vi "Autonomous Independent.vi"() -> ()   [LabVIEW 2016]
doc: "This VI is called when autonomous begins, and will automatically be terminated when autonomous ends. You can carry out timed or sensor driven robot movement independently without needing to return to the caller."
uses:
  2_8_17/Auto_Action.ctl
  <vilib>/Rock Robotics/Network Tables/NT Read Number.vi
  2_11_17/Systems/Global 1.vi
panel:
  out "In Range?":bool=TRUE
  out "Auto Mode":dbl=7.0
  in  "Auton_Modes":T2(array[cluster])=[{"Actions"=[{"Effort"=0.55, "Duration"=3.5, "Action"=enum."Nothing", "Encoder"=0.0, "Condition"=FALSE}, {"Effort"=0.0, "Duration"=0.0, "Action"=enum."Nothing", "Encoder"=0.0, "Condition"=FALSE}]}, {"Actions"=[{"Effort"=0.0, "Duration"=0.1, "Action"=enum."Gear1", "Encoder"=6.462, "Condition"=FALSE}, {"Effort"=0.0, "Duration"=0.1, "Action"=enum."Nothing", "Encoder"=0.0, "Condition"=FALSE}, {"Effort"=0.25, "Duration"=1.0, "Action"=enum."Nothing", "Encoder"=38.0, "Condition"=FALSE}, {"Effort"=0.0, "Duration"=0.1, "Action"=enum."Nothing", "Encoder"=0.0, "Condition"=FALSE}, {"Effort"=0.25, "Duration"=0.0, "Action"=enum."Nothing", "Encoder"=57.0, "Condition"=FALSE}, {"Effort"=-0.25, "Duration"=0.0, "Action"=enum."Nothing", "Encoder"=0.0, "Condition"=FALSE}, {"Effort"=1.0, "Duration"=0.0, "Action"=enum."Nothing", "Encoder"=0.0, "Condition"=FALSE}, {"Effort"=0.25, "Duration"=0.0, "Action"=enum."Nothing", "Encoder"=0.0, "Condition"=FALSE}]}, {"Actions"=[{"Effort"=0.0, "Duration"=0.1, "Action"=enum."Drive Encoder Reset", "Encoder"=0.0, "Condition"=FALSE}, {"Effort"=0.0, "Duration"=1.0, "Action"=enum."Gyro Reset", "Encoder"=0.0, "Condition"=FALSE}, {"Effort"=0.3, "Duration"=2.0, "Action"=enum."Drive", "Encoder"=88.0, "Condition"=TRUE}, {"Effort"=1.0, "Duration"=1.0, "Action"=enum."Gear0", "Encoder"=0.0, "Condition"=FALSE}, {"Effort"=1.0, "Duration"=1.0, "Action"=enum."Gear0", "Encoder"=0.0, "Condition"=FALSE}, {"Effort"=1.0, "Duration"=0.5, "Action"=enum."Nothing", "Encoder"=0.0, "Condition"=FALSE}, {"Effort"=0.0, "Duration"=0.0, "Action"=enum."Drive Encoder Reset", "Encoder"=0.0, "Condition"=FALSE}, {"Effort"=0.3, "Duration"=0.5, "Action"=enum."Nothing", "Encoder"=24.0, "Condition"=TRUE}, {"Effort"=0.0, "Duration"=0.0, "Action"=enum."Nothing", "Encoder"=0.0, "Condition"=FALSE}, {"Effort"=-0.2, "Duration"=0.75, "Action"=enum."Drive", "Encoder"=24.0, "Condition"=FALSE}, {"Effort"=0.0, "Duration"=0.0, "Action"=enum."Drive Encoder Reset", "Encoder"=0.0, "Condition"=FALSE}, {"Effort"=-0.25, "Duration"=0.0, "Action"=enum."Nothing", "Encoder"=12.0, "Condition"=FALSE}]}, {"Actions"=[{"Effort"=0.0, "Duration"=0.1, "Action"=enum."Drive Encoder Reset", "Encoder"=6.462, "Condition"=FALSE}, {"Effort"=0.0, "Duration"=0.1, "Action"=enum."Gyro Reset", "Encoder"=0.0, "Condition"=FALSE}, {"Effort"=-0.25, "Duration"=1.0, "Action"=enum."Drive", "Encoder"=6.462, "Condition"=FALSE}, {"Effort"=0.0, "Duration"=0.1, "Action"=enum."Gyro Reset", "Encoder"=0.0, "Condition"=FALSE}, {"Effort"=-0.25, "Duration"=0.0, "Action"=enum."Turn", "Encoder"=57.0, "Condition"=FALSE}, {"Effort"=-0.25, "Duration"=0.0, "Action"=enum."Drive", "Encoder"=7.5, "Condition"=FALSE}, {"Effort"=-1.0, "Duration"=0.0, "Action"=enum."Gear0", "Encoder"=0.0, "Condition"=FALSE}, {"Effort"=0.25, "Duration"=0.0, "Action"=enum."Drive", "Encoder"=3.0, "Condition"=FALSE}]}, {"Actions"=[{"Effort"=0.0, "Duration"=0.1, "Action"=enum."Drive Encoder Reset", "Encoder"=6.462, "Condition"=FALSE}, {"Effort"=0.0, "Duration"=0.1, "Action"=enum."Gyro Reset", "Encoder"=0.0, "Condition"=FALSE}, {"Effort"=-0.25, "Duration"=1.0, "Action"=enum."Drive", "Encoder"=72.0, "Condition"=FALSE}, {"Effort"=0.0, "Duration"=0.1, "Action"=enum."Gyro Reset", "Encoder"=0.0, "Condition"=FALSE}, {"Effort"=-0.25, "Duration"=2.0, "Action"=enum."Turn", "Encoder"=57.0, "Condition"=FALSE}, {"Effort"=-0.25, "Duration"=0.0, "Action"=enum."Drive", "Encoder"=36.0, "Condition"=FALSE}, {"Effort"=-1.0, "Duration"=0.0, "Action"=enum."Gear0", "Encoder"=0.0, "Condition"=FALSE}, {"Effort"=0.25, "Duration"=0.0, "Action"=enum."Drive", "Encoder"=24.0, "Condition"=FALSE}]}, {"Actions"=[{"Effort"=0.0, "Duration"=0.1, "Action"=enum."Vision Correction", "Encoder"=0.0, "Condition"=FALSE}, {"Effort"=0.0, "Duration"=0.1, "Action"=enum."Nothing", "Encoder"=0.0, "Condition"=FALSE}, {"Effort"=0.25, "Duration"=1.0, "Action"=enum."Nothing", "Encoder"=6.462, "Condition"=FALSE}, {"Effort"=1.0, "Duration"=0.1, "Action"=enum."Nothing", "Encoder"=0.0, "Condition"=FALSE}, {"Effort"=0.25, "Duration"=0.0, "Action"=enum."Nothing", "Encoder"=57.0, "Condition"=FALSE}, {"Effort"=0.25, "Duration"=0.0, "Action"=enum."Nothing", "Encoder"=7.5, "Condition"=FALSE}, {"Effort"=1.0, "Duration"=0.0, "Action"=enum."Nothing", "Encoder"=0.0, "Condition"=FALSE}, {"Effort"=-0.25, "Duration"=0.0, "Action"=enum."Nothing", "Encoder"=3.0, "Condition"=FALSE}]}, {"Actions"=[{"Effort"=0.0, "Duration"=0.1, "Action"=enum."Drive Encoder Reset", "Encoder"=0.0, "Condition"=FALSE}, {"Effort"=0.0, "Duration"=0.1, "Action"=enum."Gyro Reset", "Encoder"=0.0, "Condition"=FALSE}, {"Effort"=0.25, "Duration"=5.0, "Action"=enum."Drive", "Encoder"=60000.0, "Condition"=TRUE}, {"Effort"=0.75, "Duration"=1.0, "Action"=enum."Nothing", "Encoder"=0.0, "Condition"=FALSE}, {"Effort"=0.0, "Duration"=1.0, "Action"=enum."Nothing", "Encoder"=0.0, "Condition"=FALSE}, {"Effort"=0.0, "Duration"=0.0, "Action"=enum."Nothing", "Encoder"=0.0, "Condition"=FALSE}]}, {"Actions"=[{"Effort"=0.0, "Duration"=0.5, "Action"=enum."Drive Encoder Reset", "Encoder"=0.0, "Condition"=FALSE}, {"Effort"=0.55, "Duration"=4.25, "Action"=enum."Gyro Reset", "Encoder"=0.0, "Condition"=FALSE}, {"Effort"=0.5, "Duration"=0.0, "Action"=enum."Drive", "Encoder"=43.0, "Condition"=FALSE}, {"Effort"=0.3, "Duration"=1.3, "Action"=enum."Turn", "Encoder"=0.0, "Condition"=TRUE}, {"Effort"=0.3, "Duration"=1.0, "Action"=enum."Drive Encoder Reset", "Encoder"=12.0, "Condition"=FALSE}, {"Effort"=0.3, "Duration"=0.5, "Action"=enum."Vision Correction", "Encoder"=5.0, "Condition"=FALSE}, {"Effort"=0.3, "Duration"=1.0, "Action"=enum."Drive", "Encoder"=18.5, "Condition"=TRUE}, {"Effort"=1.0, "Duration"=0.0, "Action"=enum."Gear0", "Encoder"=0.0, "Condition"=FALSE}, {"Effort"=-0.3, "Duration"=0.0, "Action"=enum."Drive", "Encoder"=30.0, "Condition"=FALSE}, {"Effort"=-0.3, "Duration"=1.3, "Action"=enum."Turn", "Encoder"=0.0, "Condition"=FALSE}, {"Effort"=0.4, "Duration"=0.0, "Action"=enum."Drive", "Encoder"=10.0, "Condition"=FALSE}]}, {"Actions"=[{"Effort"=0.0, "Duration"=0.0, "Action"=enum."Nothing", "Encoder"=0.0, "Condition"=FALSE}, {"Effort"=0.0, "Duration"=0.0, "Action"=enum."Nothing", "Encoder"=0.0, "Condition"=FALSE}, {"Effort"=0.0, "Duration"=0.0, "Action"=enum."Gyro Reset", "Encoder"=0.0, "Condition"=FALSE}]}]
  # "Nothing"
  # "Boiler Right Right side gear"
  # "Middle Gear"
  # "Boiler Right Left Side Gear"
  # "Boiler Left RightSide Gear"
  # "Boiler Left Left Side Gear"
  # "Drive"
  # "Vision Correction"
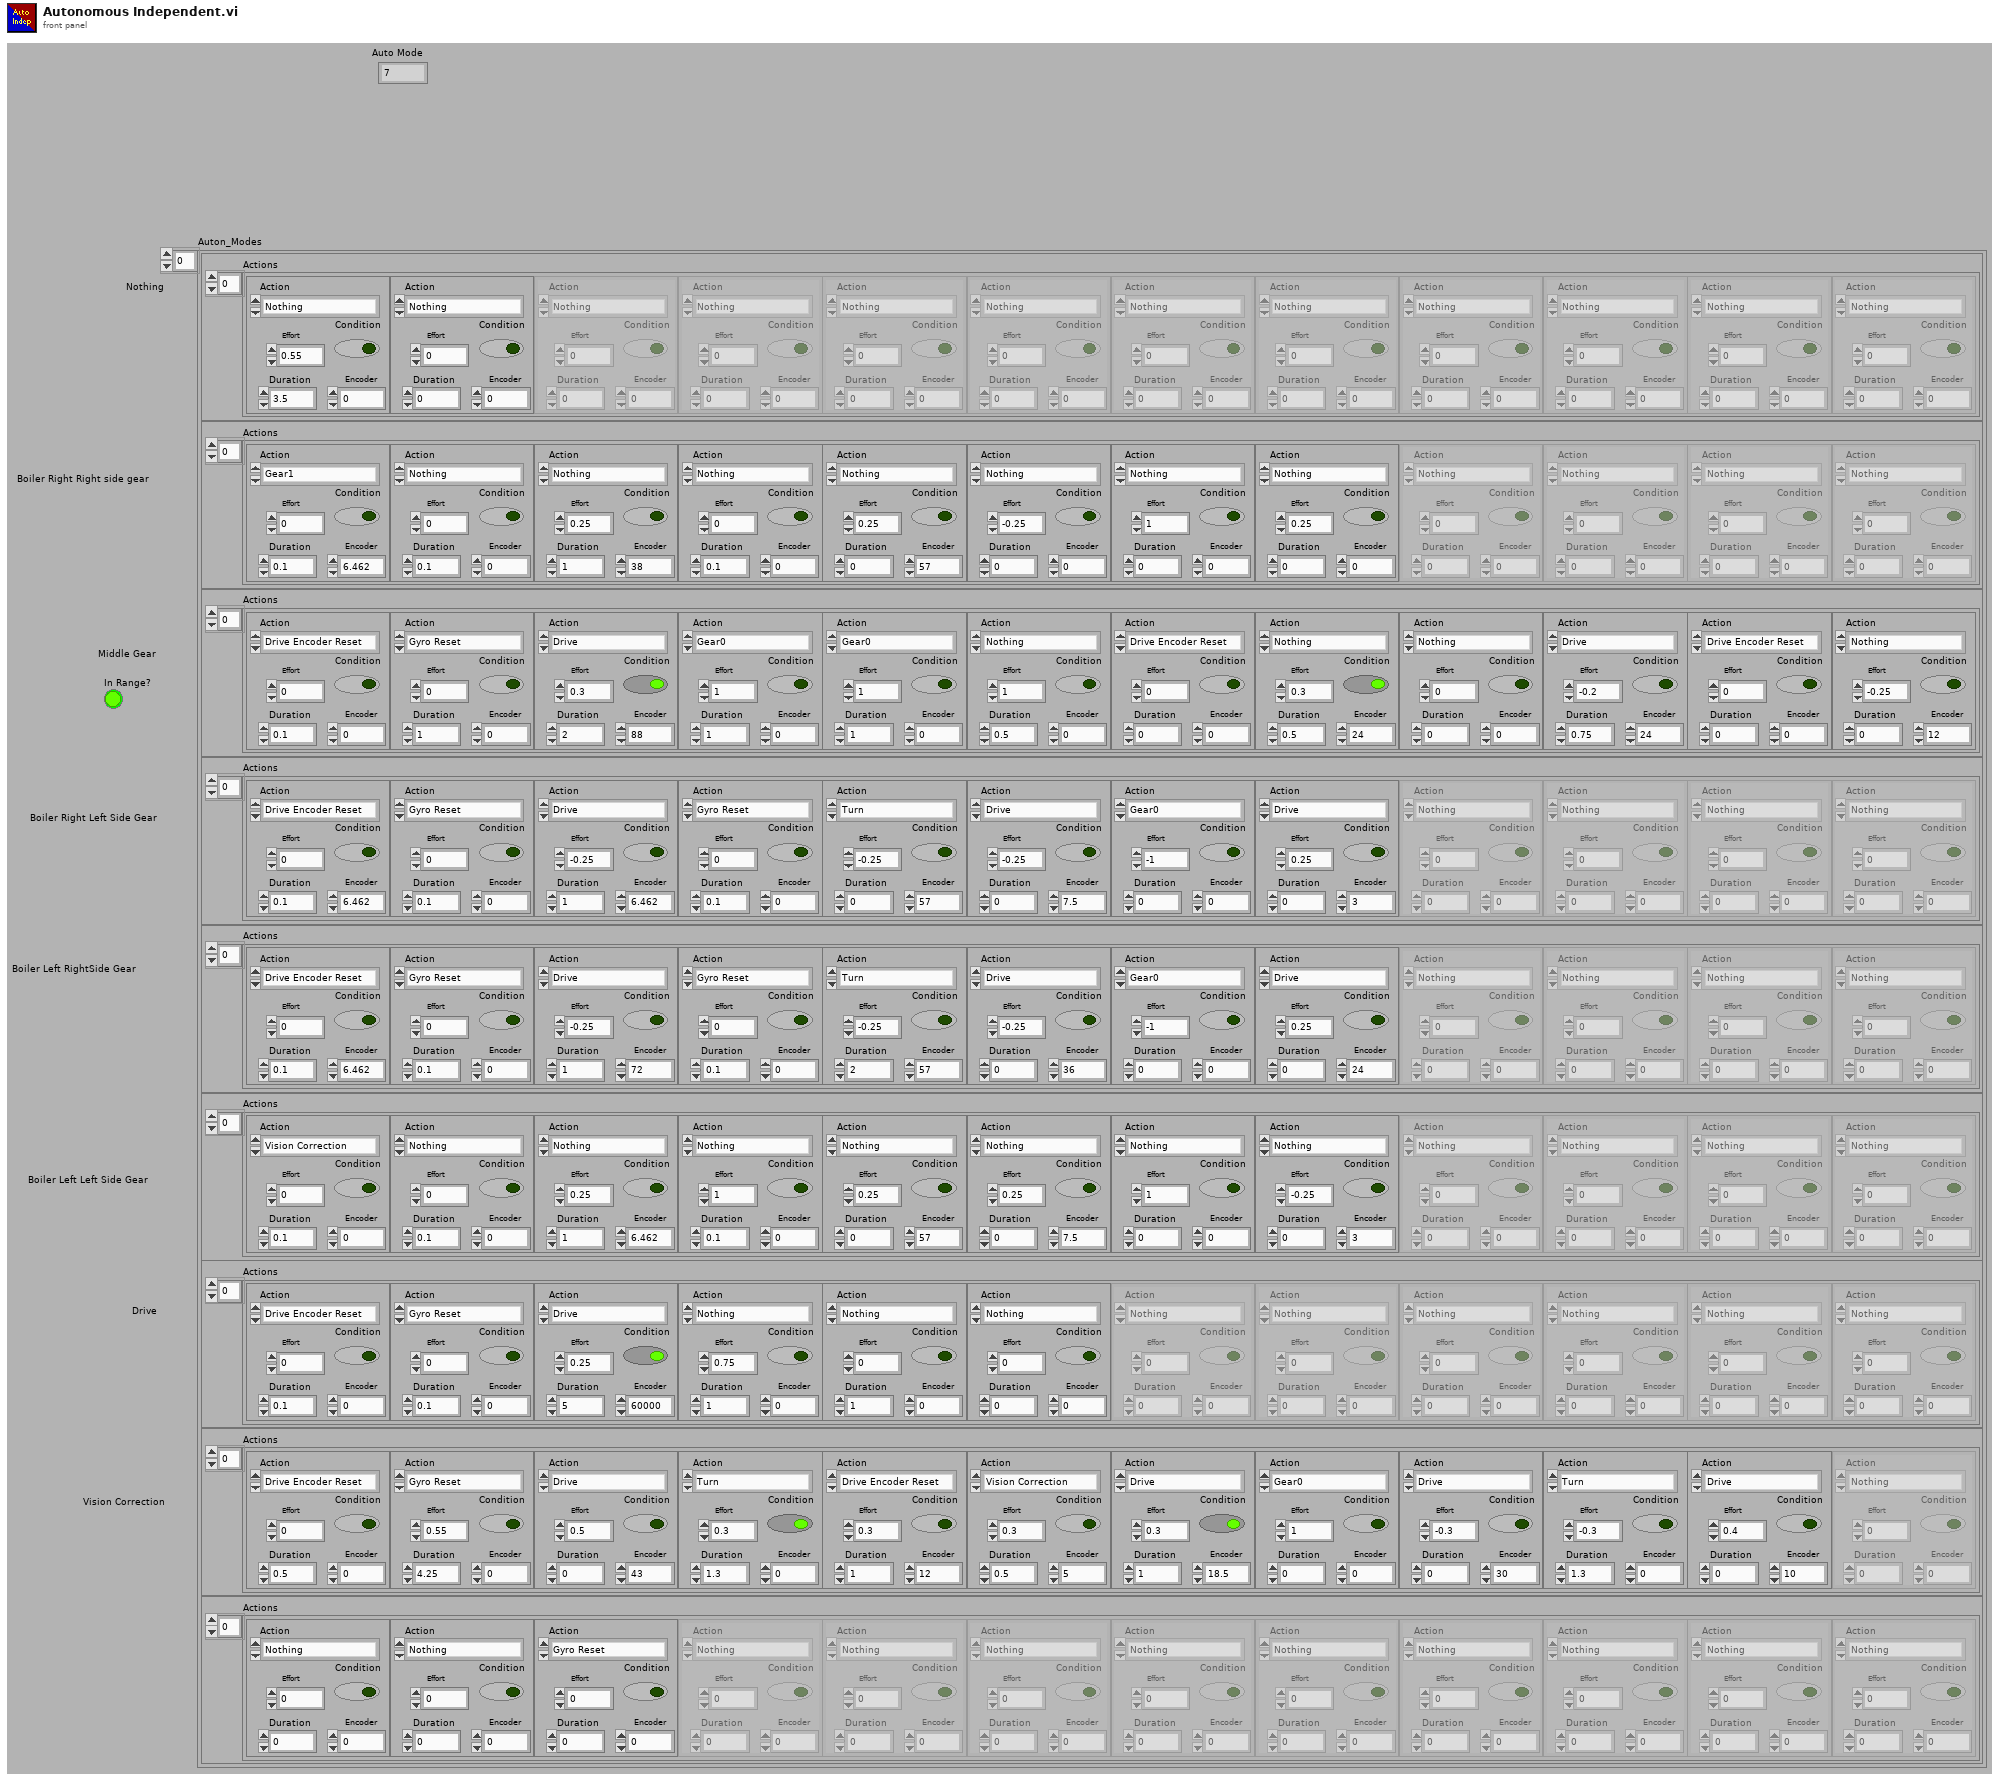
[diagram p1: front panel]
types:
  T1 = typedef "Auto_Action.ctl" = enum16{"Nothing", "Drive", "Vision Correction", "Turn", "Gear0", "Gear1", "Climb", "Intake", "Index", "Shoot", "Test", "Drive Encoder Reset", "Gyro Reset"}
  T2 = cluster{"Actions":cluster{"Effort":dbl, "Duration":dbl, "Action":T1, "Encoder":dbl, "Condition":bool}[]}[]
  T3 = cluster{"Actions":cluster{"Effort":dbl, "Duration":dbl, "Action":T1, "Encoder":dbl, "Condition":bool}[]}
  T4 = cluster{"Effort":dbl, "Duration":dbl, "Action":T1, "Encoder":dbl, "Condition":bool}[]
  T5 = typedef "WPI_MotorControlDeviceRef.ctl" = cluster{"DeviceStatus":errorcluster, "Type":T6, "PWM":cluster{"PWM Channel":T7, "DeadBand":T8}, "CAN":cluster{"Device Number":u8, "SetOutput VI Ref":variant, "GetOutput VI Ref":variant, "Enable VI Ref":variant, "Disable VI Ref":variant, "Data":variant}, "Invert":bool}
  T6 = typedef "WPI_MotorControlType.ctl" = enum16{"PWM", "CAN"}
  T7 = typedef "FPGA_DIOPWMChannel.ctl" = enum8{"PWM 0", "PWM 1", "PWM 2", "PWM 3", "PWM 4", "PWM 5", "PWM 6", "PWM 7", "PWM 8", "PWM 9", "PWM MXP 0", "PWM MXP 1", "PWM MXP 2", "PWM MXP 3", "PWM MXP 4", "PWM MXP 5", "PWM MXP 6", "PWM MXP 7", "PWM MXP 8", "PWM MXP 9", "Invalid"}
  T8 = typedef "WPI_PWMDeadband.ctl" = cluster{"Name":string, "maxPositivePwm":i32, "minPositivePwm":i32, "centerPwm":i32, "maxNegativePwm":i32, "minNegativePwm":i32, "angularRange":u16}
  T9 = typedef "WPI_CANTalonSRX_GlobalStatus.ctl" = cluster{"Applied Throttle":dbl, "Module Enabled":bool, "CAN Error":errorcluster, "Closed Loop Error":dbl, "Forward Limit Switch Closed":bool, "Reverse Limit Switch Closed":bool, "Sensor Position":dbl, "Sensor Velocity":dbl, "Current":dbl, "Sticky Fault - Over Temp":bool, "Sticky Fault - Under Voltage":bool, "Sticky Fault - Forward Limit":bool, "Sticky Fault - Reverse Limit":bool, "Sticky Fault - Forward Soft Limit":bool, "Sticky Fault - Reverse Soft Limit":bool, "Brake is Enabled":bool, "Encoder Position":dbl, "Encoder Velocity":dbl, "Encoder Index Count":dbl, "Encoder A Pin State":bool, "Encoder B Pin State":bool, "Encoder Index Pin State":bool, "Analog In":dbl, "Analog In Velocity":dbl, "Temperature (C)":dbl, "Battery Voltage":dbl, "Control 5 Is Supported":bool, "Current Profile Slot Select":dbl, "Pos Div 8":bool, "Vel Div 4":bool, "Pulse Width Position":i32, "Pulse Width Velocity":i32, "Pulse Width Rise To Rise (us)":i32, "Pulse Width Rise To Fall (us)":i32, "Mot Prof Active Is Under Run":bool, "Mot Prof Active Has Under Run":bool, "Mot Prof Active Is Last":bool, "Mot Prof Active Velocity Only":bool, "Mot Prof Active Is Valid":bool, "Mot Prof Buffer Is Full":bool, "Mot Prof Active Profile Slot Select":i32, "Mot Prof NextID":i32, "Mot Prof Count":i32, "Mot Prof Active Velocity":dbl, "Mot Prof Active Position":dbl, "Mot Prof Output Enable":i32}
  T10 = typedef "WPI_GyroDevRef.ctl" = cluster{"DevStatus":errorcluster, "Analog Channel":T11, "Offset":dbl, "Gain (VoltsPerDegree/Second)":dbl, "Gyro Type":enum16{"Analog", "XRS450"}, "Handle":i32, "SPI Bus":T12, "Device Found":bool, "Sample Rate":dbl, "Calibrate On Open":bool}
  T11 = typedef "FPGA_AIChannel.ctl" = enum8{"AI 0", "AI 1", "AI 2", "AI 3", "AI MXP 0", "AI MXP 1", "AI MXP 2", "AI MXP 3", "Invalid"}
  T12 = typedef "spi_bus.ctl" = enum16{"SPI On-Board, CS0", "SPI On-Board, CS1", "SPI On-Board, CS2", "SPI On-Board, CS3", "SPI MXP", "Invalid"}
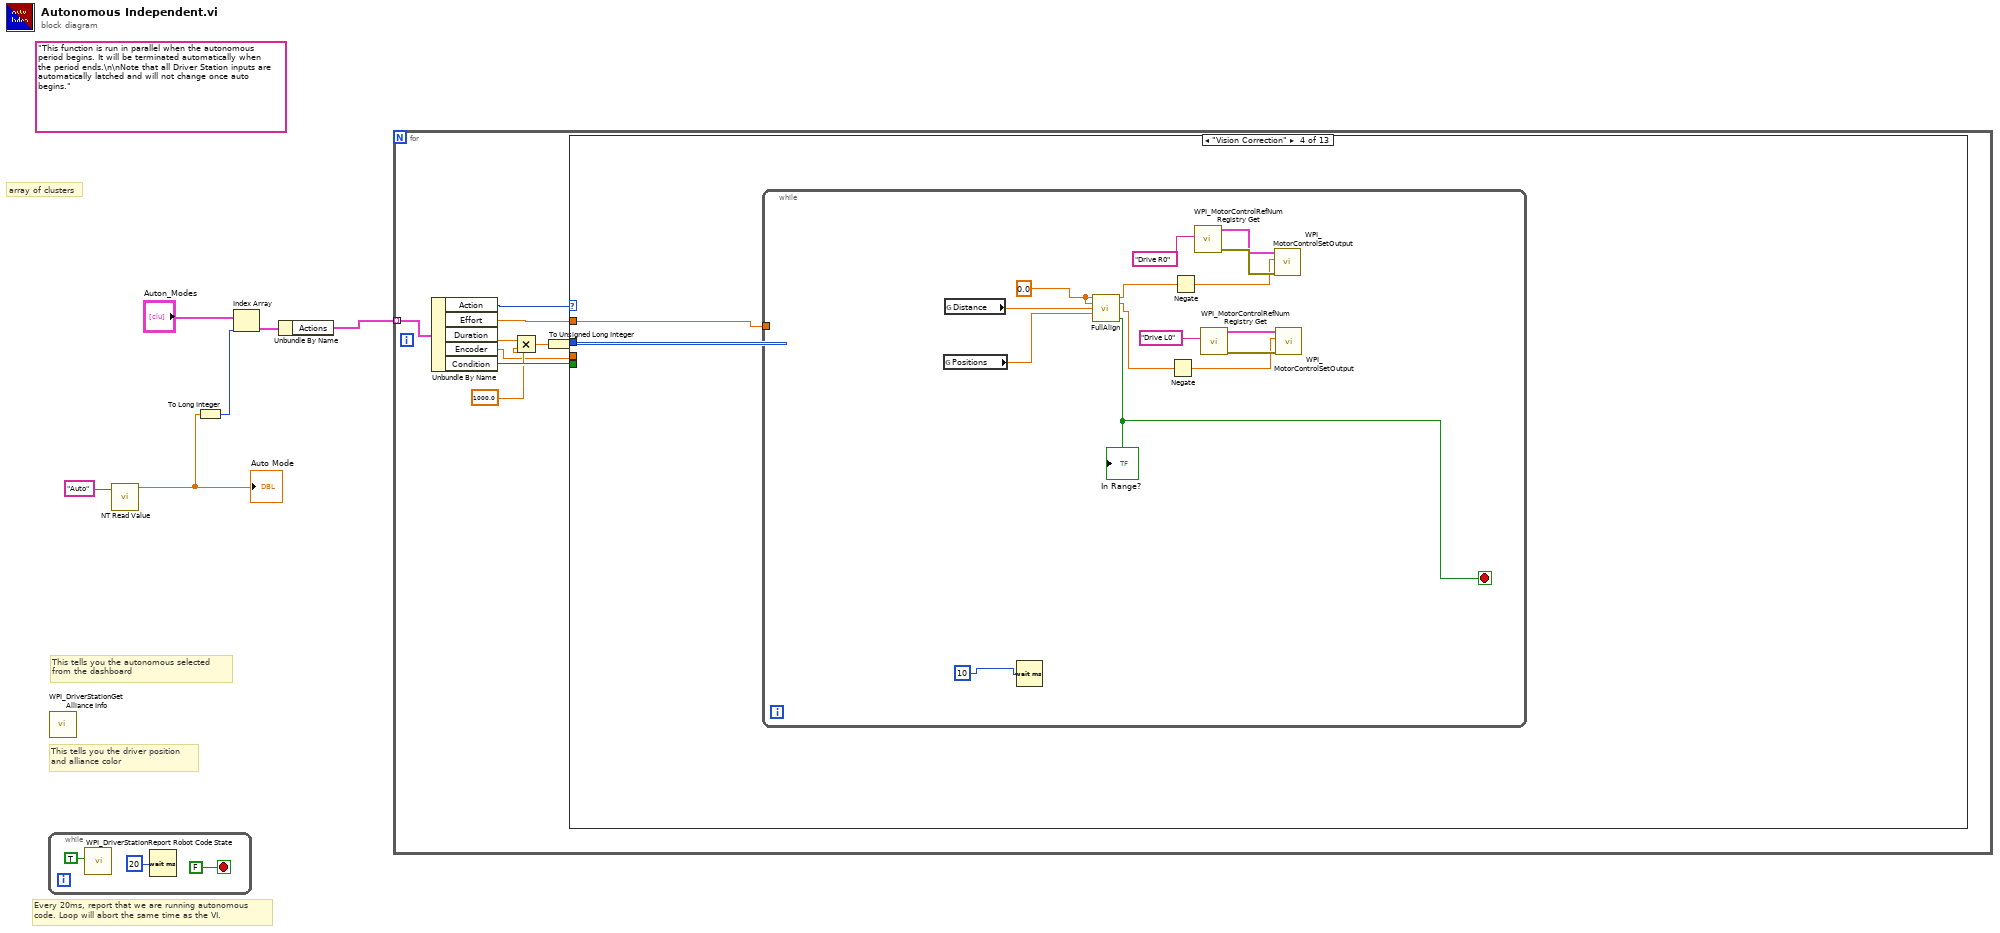
[diagram p0: block diagram]
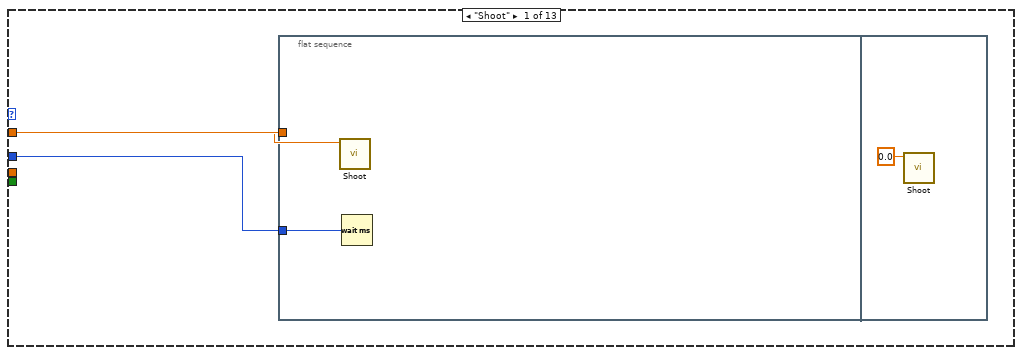
[diagram p2: hidden frame]
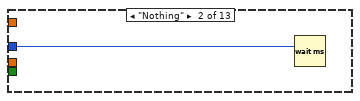
[diagram p3: hidden frame]
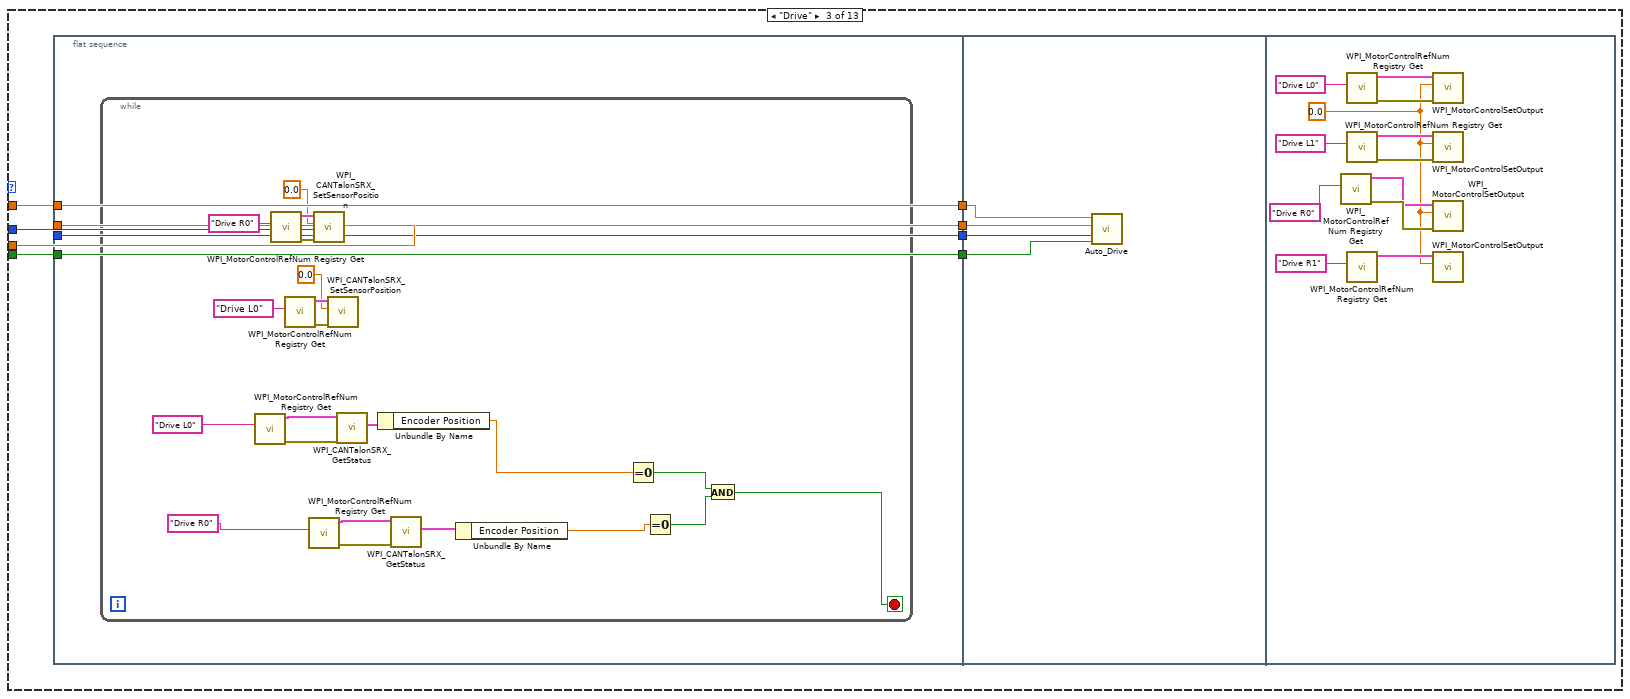
[diagram p4: hidden frame]
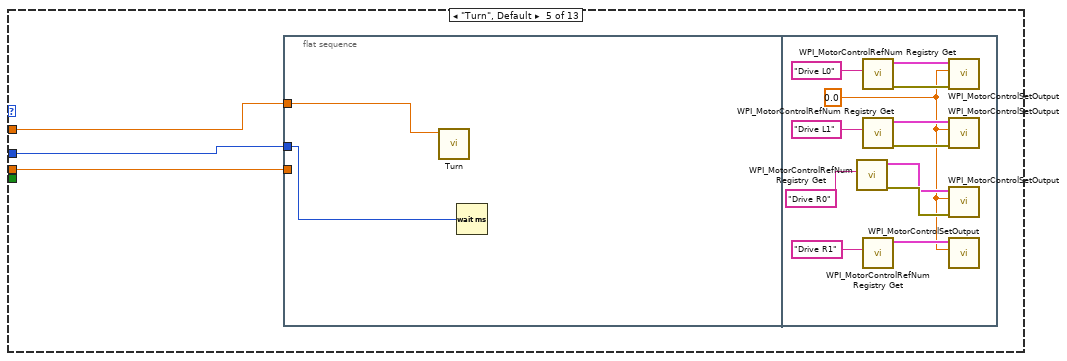
[diagram p5: hidden frame]
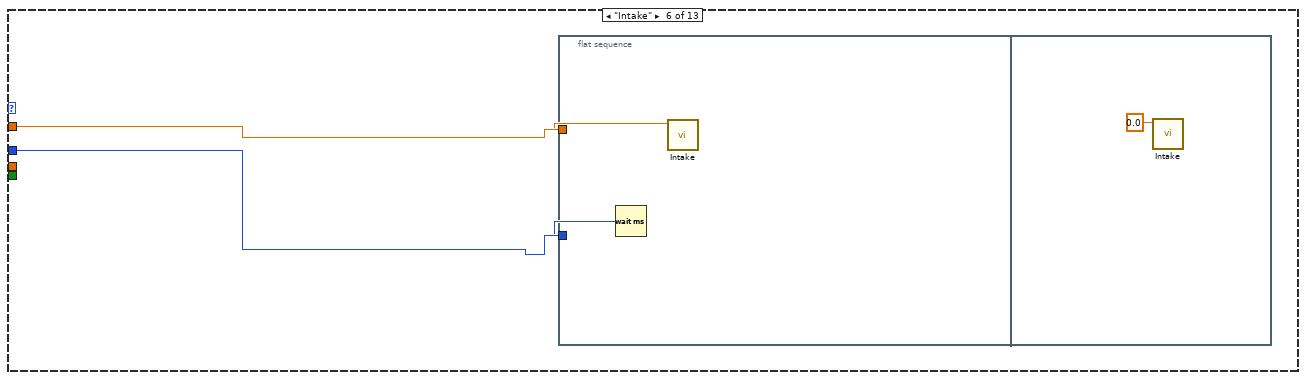
[diagram p6: hidden frame]
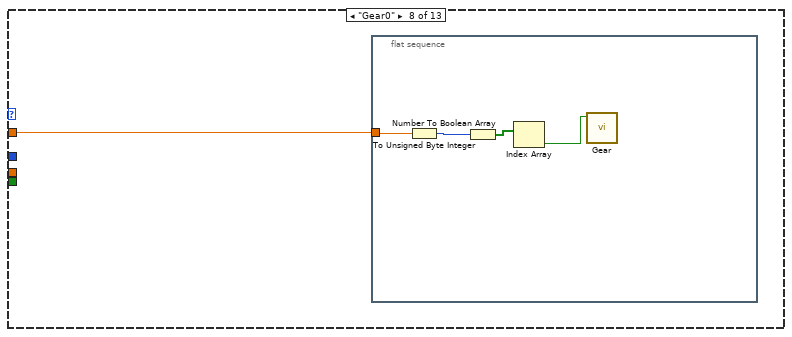
[diagram p8: hidden frame]
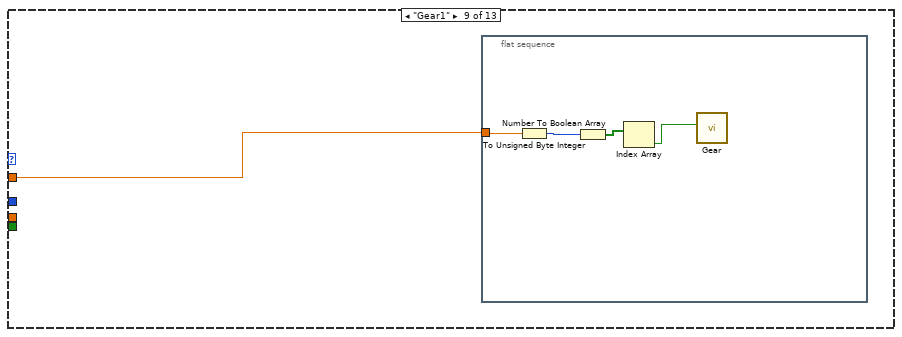
[diagram p9: hidden frame]
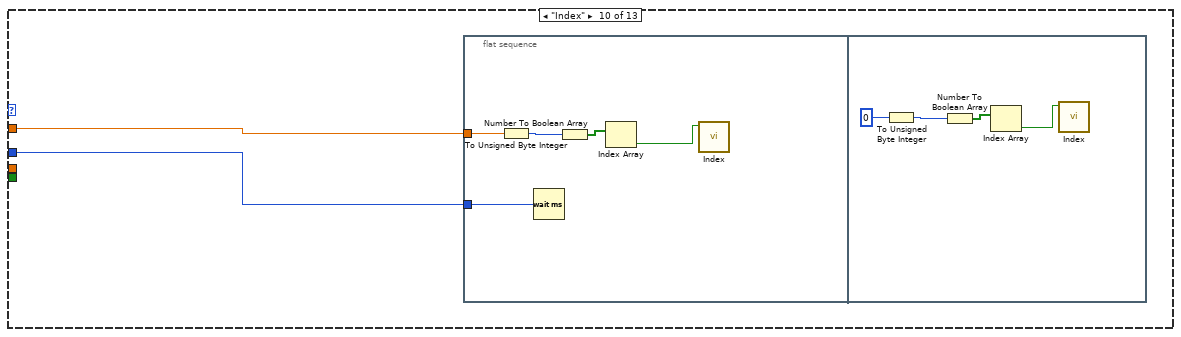
[diagram p10: hidden frame]
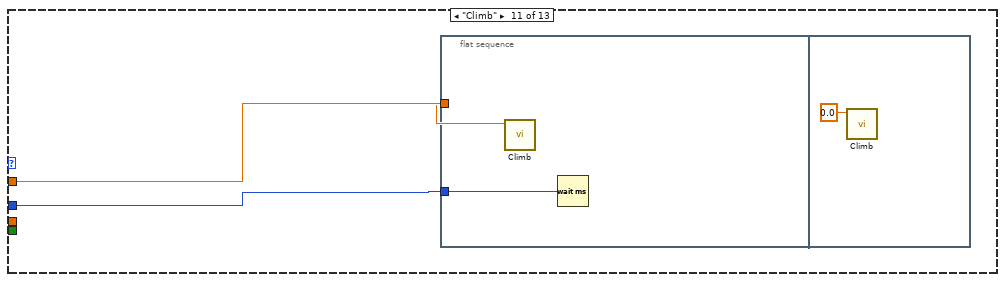
[diagram p11: hidden frame]
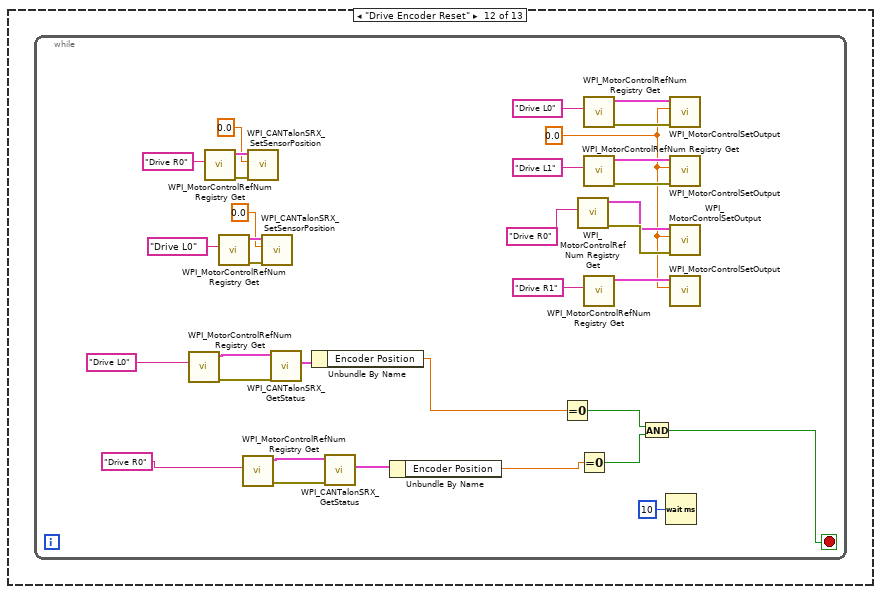
[diagram p12: hidden frame]
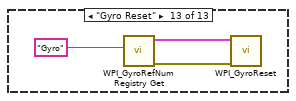
[diagram p13: hidden frame]
diagram:
  (unwired) "This function is run in parallel when the autonomous period begins. It will be terminated automatically when the period ends.\n\nNote that all Driver Station inputs are automatically latched and will not change once auto begins."
  # "This tells you the autonomous selected\nfrom the dashboard"
  # "array of clusters"
  # "Every 20ms, report that we are running autonomous\ncode. Loop will abort the same time as the VI."
  # "This tells you the driver position\nand alliance color"
  n1 = while {
    stop <- FALSE stop-if-true
    n2 = call <vilib>:"WPI_DriverStationReport Robot Code State.vi"("Autonomous"=TRUE) -> ()  [unwired: 10 in, 1 out]
    n3 = Wait (ms)(milliseconds to wait=u32 20) -> ()  [unwired: 1 out]
  }
  n4 = call <vilib>:"WPI_DriverStationGet Alliance Info.vi"() -> ()  [unwired: 12 out]
  n5 = call-poly <vilib>:"NT Read Value.vi"("Name"="Auto") -> ("Numeric"=w1:dbl)  [unwired: 9 in, 1 out]
  "Auto Mode" <- w1
  n6 = To Long Integer(number=w1) -> (32bit integer=w3:i32)
  n7 = Index Array(array="Auton_Modes", index=w3) -> (element=w5:T3)
  n8 = Unbundle By Name(w5) -> ("Actions"=w6:T4)
  n9 = for {
    tunnel: w6 -> [w18] mode=indexing
    n10 = Unbundle By Name(w18) -> ("Action"=w17:T1, "Effort"=w16:dbl, "Duration"=w15:dbl, "Encoder"=w10:dbl, "Condition"=w12:bool)
    n11 = Multiply(x=w15, y=1000.0) -> (x*y=w14:dbl)
    n12 = To Unsigned Long Integer(number=w14) -> (unsigned 32bit integer=w13:u32)
    n13 = case shown="\"Vision Correction\"" w17 {
      tunnel: w16 -> [w20 _ w32 w74 w92 w108 _ w112 w117 w122 w134 _ _]
      tunnel: w13 -> [w19 w24 w31 _ w91 w107 _ _ _ w123 w133 _ _]
      tunnel: w12 -> [_ _ w30 _ _ _ _ _ _ _ _ _ _]
      tunnel: w10 -> [_ _ w29 _ w90 _ _ _ _ _ _ _ _]
      frame "Shoot" {
        n14 = flat-sequence {
          tunnel: w20 -> [w22]
          tunnel: w19 -> [w21]
          frame #0 {
            n15 = call "Shoot.vi"("Set RPM"=w22) -> ()  [unwired: 11 in]
            n16 = Wait (ms)(milliseconds to wait=w21) -> ()  [unwired: 1 out]
          }
          frame #1 {
            n17 = call "Shoot.vi"("Set RPM"=0.0 ("Effort")) -> ()  [unwired: 11 in]
          }
        }
      }
      frame "Nothing" {
        n18 = Wait (ms)(milliseconds to wait=w24) -> ()  [unwired: 1 out]
      }
      frame "Drive" {
        n19 = flat-sequence {
          tunnel: w29 -> [w33]
          tunnel: w30 -> [w34]
          tunnel: w31 -> [w35]
          tunnel: w32 -> [w36]
          tunnel: [w36] -> w28
          tunnel: [w35] -> w27
          tunnel: [w34] -> w26
          tunnel: [w33] -> w25
          tunnel: w28 -> [w61]
          tunnel: w27 -> [w60]
          tunnel: w26 -> [w59]
          tunnel: w25 -> [w58]
          frame #0 {
            n20 = while {
              stop <- w37 stop-if-true
              n21 = call <vilib>:"WPI_MotorControlRefNum Registry Get.vi"("refnum name"="Drive L0") -> ("error out"=w47:errorcluster, "MotorControlDevRef"=w42:T5)  [unwired: 9 in]
              n22 = call <vilib>:"WPI_MotorControlRefNum Registry Get.vi"("refnum name"="Drive R0") -> ("error out"=w52:errorcluster, "MotorControlDevRef"=w51:T5)  [unwired: 9 in]
              n23 = call <vilib>:"WPI_MotorControlRefNum Registry Get.vi"("refnum name"="Drive L0") -> ("error out"=w54:errorcluster, "MotorControlDevRef"=w55:T5)  [unwired: 9 in]
              n24 = call <vilib>:"WPI_MotorControlRefNum Registry Get.vi"("refnum name"="Drive R0") -> ("error out"=w44:errorcluster, "MotorControlDevRef"=w43:T5)  [unwired: 9 in]
              n25 = call <vilib>:"WPI_CANTalonSRX_SetSensorPosition.vi"("error in (no error)"=w52, "New Sensor Position"=0.0, "CAN Talon SRX Ref"=w51) -> ()  [unwired: 7 in, 2 out]
              n26 = call <vilib>:"WPI_CANTalonSRX_SetSensorPosition.vi"("error in (no error)"=w54, "New Sensor Position"=0.0, "CAN Talon SRX Ref"=w55) -> ()  [unwired: 7 in, 2 out]
              n27 = call <vilib>:"WPI_CANTalonSRX_GetStatus.vi"("error in (no error)"=w47, "CAN Talon SRX Ref"=w42) -> ("Talon SRX Status"=w45:T9)  [unwired: 7 in, 2 out]
              n28 = Unbundle By Name(w45) -> ("Encoder Position"=w40:dbl)
              n29 = call <vilib>:"WPI_CANTalonSRX_GetStatus.vi"("error in (no error)"=w44, "CAN Talon SRX Ref"=w43) -> ("Talon SRX Status"=w46:T9)  [unwired: 7 in, 2 out]
              n30 = Unbundle By Name(w46) -> ("Encoder Position"=w41:dbl)
              n31 = Equal To 0?(x=w40) -> (x = 0?=w39:bool)
              n32 = Equal To 0?(x=w41) -> (x = 0?=w38:bool)
              n33 = And(x=w39, y=w38) -> (x .and. y?=w37:bool)
            }
          }
          frame #1 {
            n34 = call "Auto_Drive.vi"("Timer?"=w59, "Duration"=w60, "distance"=w58, "Drive Effort"=w61) -> ()  [unwired: 8 in]
          }
          frame #2 {
            w62 = 0.0 ("Drive L")
            n35 = call <vilib>:"WPI_MotorControlRefNum Registry Get.vi"("refnum name"="Drive R0") -> ("error out"=w67:errorcluster, "MotorControlDevRef"=w63:T5)  [unwired: 9 in]
            n36 = call <vilib>:"WPI_MotorControlRefNum Registry Get.vi"("refnum name"="Drive L0") -> ("error out"=w68:errorcluster, "MotorControlDevRef"=w69:T5)  [unwired: 9 in]
            n37 = call <vilib>:"WPI_MotorControlRefNum Registry Get.vi"("refnum name"="Drive L1") -> ("error out"=w72:errorcluster, "MotorControlDevRef"=w71:T5)  [unwired: 9 in]
            n38 = call <vilib>:"WPI_MotorControlRefNum Registry Get.vi"("refnum name"="Drive R1") -> ("MotorControlDevRef"=w65:T5)  [unwired: 9 in, 1 out]
            n39 = call <vilib>:"WPI_MotorControlSetOutput.vi"("error in (no error)"=w68, "Output"=w62, "MotorControlDevRef"=w69) -> ()  [unwired: 6 in, 3 out]
            n40 = call <vilib>:"WPI_MotorControlSetOutput.vi"("error in (no error)"=w72, "Output"=w62, "MotorControlDevRef"=w71) -> ()  [unwired: 6 in, 3 out]
            n41 = call <vilib>:"WPI_MotorControlSetOutput.vi"("error in (no error)"=w67, "Output"=w62, "MotorControlDevRef"=w63) -> ()  [unwired: 6 in, 3 out]
            n42 = call <vilib>:"WPI_MotorControlSetOutput.vi"("Output"=w62, "MotorControlDevRef"=w65) -> ()  [unwired: 7 in, 3 out]
          }
        }
      }
      frame "Vision Correction" {
        n43 = while {
          tunnel: w74 -> [_]
          stop <- w76 stop-if-true
          w83 = 0.0
          n44 = global read "Global 1.vi" "Positions"() -> (w81:dbl)
          n45 = global read "Global 1.vi" "Distance"() -> (w82:dbl)
          n46 = Wait (ms)(milliseconds to wait=u32 10 ("millisecond timer value")) -> ()  [unwired: 1 out]
          n47 = call "FullAlign.vi"("Joystick 0"=w83, "Joystick 1"=w83, "Distance"=w82, "Angle"=w81) -> ("Right Motor"=w79:dbl, "Left Motor"=w80:dbl, "In Range?"=w76:bool)  [unwired: 9 in]
          "In Range?" <- w76
          n48 = Negate(x=w80) -> (-x=w77:dbl)
          n49 = Negate(x=w79) -> (-x=w78:dbl)
          n50 = call <vilib>:"WPI_MotorControlRefNum Registry Get.vi"("refnum name"="Drive R0") -> ("error out"=w86:errorcluster, "MotorControlDevRef"=w84:T5)  [unwired: 9 in]
          n51 = call <vilib>:"WPI_MotorControlRefNum Registry Get.vi"("refnum name"="Drive L0") -> ("error out"=w87:errorcluster, "MotorControlDevRef"=w88:T5)  [unwired: 9 in]
          n52 = call <vilib>:"WPI_MotorControlSetOutput.vi"("error in (no error)"=w86, "Output"=w78, "MotorControlDevRef"=w84) -> ()  [unwired: 6 in, 3 out]
          n53 = call <vilib>:"WPI_MotorControlSetOutput.vi"("error in (no error)"=w87, "Output"=w77, "MotorControlDevRef"=w88) -> ()  [unwired: 6 in, 3 out]
        }
      }
      frame "Turn", Default {
        n54 = flat-sequence {
          tunnel: w92 -> [w94]
          tunnel: w91 -> [w93]
          tunnel: w90 -> [_]
          frame #0 {
            n55 = call "Turn.vi"("Effort"=w94) -> ()  [unwired: 11 in]
            n56 = Wait (ms)(milliseconds to wait=w93) -> ()  [unwired: 1 out]
          }
          frame #1 {
            w95 = 0.0 ("Drive L")
            n57 = call <vilib>:"WPI_MotorControlRefNum Registry Get.vi"("refnum name"="Drive R0") -> ("error out"=w100:errorcluster, "MotorControlDevRef"=w96:T5)  [unwired: 9 in]
            n58 = call <vilib>:"WPI_MotorControlRefNum Registry Get.vi"("refnum name"="Drive L0") -> ("error out"=w101:errorcluster, "MotorControlDevRef"=w102:T5)  [unwired: 9 in]
            n59 = call <vilib>:"WPI_MotorControlRefNum Registry Get.vi"("refnum name"="Drive L1") -> ("error out"=w105:errorcluster, "MotorControlDevRef"=w104:T5)  [unwired: 9 in]
            n60 = call <vilib>:"WPI_MotorControlRefNum Registry Get.vi"("refnum name"="Drive R1") -> ("MotorControlDevRef"=w98:T5)  [unwired: 9 in, 1 out]
            n61 = call <vilib>:"WPI_MotorControlSetOutput.vi"("error in (no error)"=w101, "Output"=w95, "MotorControlDevRef"=w102) -> ()  [unwired: 6 in, 3 out]
            n62 = call <vilib>:"WPI_MotorControlSetOutput.vi"("error in (no error)"=w105, "Output"=w95, "MotorControlDevRef"=w104) -> ()  [unwired: 6 in, 3 out]
            n63 = call <vilib>:"WPI_MotorControlSetOutput.vi"("error in (no error)"=w100, "Output"=w95, "MotorControlDevRef"=w96) -> ()  [unwired: 6 in, 3 out]
            n64 = call <vilib>:"WPI_MotorControlSetOutput.vi"("Output"=w95, "MotorControlDevRef"=w98) -> ()  [unwired: 7 in, 3 out]
          }
        }
      }
      frame "Intake" {
        n65 = flat-sequence {
          tunnel: w108 -> [w110]
          tunnel: w107 -> [w109]
          frame #0 {
            n66 = Wait (ms)(milliseconds to wait=w109) -> ()  [unwired: 1 out]
            n67 = call "Intake.vi"("Effort"=w110) -> ()  [unwired: 11 in]
          }
          frame #1 {
            n68 = call "Intake.vi"("Effort"=0.0) -> ()  [unwired: 11 in]
          }
        }
      }
      frame "Test" {
      }
      frame "Gear0" {
        n69 = flat-sequence {
          tunnel: w112 -> [w116]
          frame #0 {
            n70 = To Unsigned Byte Integer(number=w116) -> (unsigned 8bit integer=w115:u8)
            n71 = Number To Boolean Array(number=w115) -> (Boolean array=w114:bool[])
            n72 = Index Array(array=w114) -> (element=w113:bool)  [unwired: 1 in]
            n73 = call "Gear.vi"("Gear0?"=w113) -> ()  [unwired: 11 in]
          }
        }
      }
      frame "Gear1" {
        n74 = flat-sequence {
          tunnel: w117 -> [w121]
          frame #0 {
            n75 = To Unsigned Byte Integer(number=w121) -> (unsigned 8bit integer=w120:u8)
            n76 = Number To Boolean Array(number=w120) -> (Boolean array=w119:bool[])
            n77 = Index Array(array=w119) -> (element=w118:bool)  [unwired: 1 in]
            n78 = call "Gear.vi"("Gear1?"=w118) -> ()  [unwired: 11 in]
          }
        }
      }
      frame "Index" {
        n79 = flat-sequence {
          tunnel: w123 -> [w125]
          tunnel: w122 -> [w124]
          frame #0 {
            n80 = To Unsigned Byte Integer(number=w124) -> (unsigned 8bit integer=w128:u8)
            n81 = Wait (ms)(milliseconds to wait=w125) -> ()  [unwired: 1 out]
            n82 = Number To Boolean Array(number=w128) -> (Boolean array=w127:bool[])
            n83 = Index Array(array=w127) -> (element=w126:bool)  [unwired: 1 in]
            n84 = call "Index.vi"("Index?"=w126) -> ()  [unwired: 11 in]
          }
          frame #1 {
            n85 = To Unsigned Byte Integer(number=u8 0) -> (unsigned 8bit integer=w131:u8)
            n86 = Number To Boolean Array(number=w131) -> (Boolean array=w132:bool[])
            n87 = Index Array(array=w132) -> (element=w129:bool)  [unwired: 1 in]
            n88 = call "Index.vi"("Index?"=w129) -> ()  [unwired: 11 in]
          }
        }
      }
      frame "Climb" {
        n89 = flat-sequence {
          tunnel: w134 -> [w136]
          tunnel: w133 -> [w135]
          frame #0 {
            n90 = call "Climb.vi"("Effort"=w136) -> ()  [unwired: 11 in]
            n91 = Wait (ms)(milliseconds to wait=w135) -> ()  [unwired: 1 out]
          }
          frame #1 {
            n92 = call "Climb.vi"("Effort"=0.0) -> ()  [unwired: 11 in]
          }
        }
      }
      frame "Drive Encoder Reset" {
        n93 = while {
          stop <- w151 stop-if-true
          w138 = 0.0 ("Drive L")
          n94 = call <vilib>:"WPI_MotorControlRefNum Registry Get.vi"("refnum name"="Drive L0") -> ("error out"=w161:errorcluster, "MotorControlDevRef"=w156:T5)  [unwired: 9 in]
          n95 = call <vilib>:"WPI_MotorControlRefNum Registry Get.vi"("refnum name"="Drive R0") -> ("error out"=w166:errorcluster, "MotorControlDevRef"=w165:T5)  [unwired: 9 in]
          n96 = call <vilib>:"WPI_MotorControlRefNum Registry Get.vi"("refnum name"="Drive L0") -> ("error out"=w168:errorcluster, "MotorControlDevRef"=w169:T5)  [unwired: 9 in]
          n97 = call <vilib>:"WPI_MotorControlRefNum Registry Get.vi"("refnum name"="Drive R0") -> ("error out"=w158:errorcluster, "MotorControlDevRef"=w157:T5)  [unwired: 9 in]
          n98 = call <vilib>:"WPI_CANTalonSRX_SetSensorPosition.vi"("error in (no error)"=w166, "New Sensor Position"=0.0, "CAN Talon SRX Ref"=w165) -> ()  [unwired: 7 in, 2 out]
          n99 = call <vilib>:"WPI_CANTalonSRX_SetSensorPosition.vi"("error in (no error)"=w168, "New Sensor Position"=0.0, "CAN Talon SRX Ref"=w169) -> ()  [unwired: 7 in, 2 out]
          n100 = call <vilib>:"WPI_CANTalonSRX_GetStatus.vi"("error in (no error)"=w161, "CAN Talon SRX Ref"=w156) -> ("Talon SRX Status"=w159:T9)  [unwired: 7 in, 2 out]
          n101 = Unbundle By Name(w159) -> ("Encoder Position"=w154:dbl)
          n102 = call <vilib>:"WPI_CANTalonSRX_GetStatus.vi"("error in (no error)"=w158, "CAN Talon SRX Ref"=w157) -> ("Talon SRX Status"=w160:T9)  [unwired: 7 in, 2 out]
          n103 = Unbundle By Name(w160) -> ("Encoder Position"=w155:dbl)
          n104 = Equal To 0?(x=w154) -> (x = 0?=w153:bool)
          n105 = call <vilib>:"WPI_MotorControlRefNum Registry Get.vi"("refnum name"="Drive R0") -> ("error out"=w143:errorcluster, "MotorControlDevRef"=w139:T5)  [unwired: 9 in]
          n106 = Equal To 0?(x=w155) -> (x = 0?=w152:bool)
          n107 = call <vilib>:"WPI_MotorControlRefNum Registry Get.vi"("refnum name"="Drive L0") -> ("error out"=w144:errorcluster, "MotorControlDevRef"=w145:T5)  [unwired: 9 in]
          n108 = call <vilib>:"WPI_MotorControlRefNum Registry Get.vi"("refnum name"="Drive L1") -> ("error out"=w148:errorcluster, "MotorControlDevRef"=w147:T5)  [unwired: 9 in]
          n109 = call <vilib>:"WPI_MotorControlRefNum Registry Get.vi"("refnum name"="Drive R1") -> ("MotorControlDevRef"=w141:T5)  [unwired: 9 in, 1 out]
          n110 = And(x=w153, y=w152) -> (x .and. y?=w151:bool)
          n111 = Wait (ms)(milliseconds to wait=u32 10) -> ()  [unwired: 1 out]
          n112 = call <vilib>:"WPI_MotorControlSetOutput.vi"("error in (no error)"=w144, "Output"=w138, "MotorControlDevRef"=w145) -> ()  [unwired: 6 in, 3 out]
          n113 = call <vilib>:"WPI_MotorControlSetOutput.vi"("error in (no error)"=w148, "Output"=w138, "MotorControlDevRef"=w147) -> ()  [unwired: 6 in, 3 out]
          n114 = call <vilib>:"WPI_MotorControlSetOutput.vi"("error in (no error)"=w143, "Output"=w138, "MotorControlDevRef"=w139) -> ()  [unwired: 6 in, 3 out]
          n115 = call <vilib>:"WPI_MotorControlSetOutput.vi"("Output"=w138, "MotorControlDevRef"=w141) -> ()  [unwired: 7 in, 3 out]
        }
      }
      frame "Gyro Reset" {
        n116 = call <vilib>:"WPI_GyroRefNum Registry Get.vi"("refnum name"="Gyro") -> ("error out"=w173:errorcluster, "GyroDevRef"=w174:T10)  [unwired: 9 in]
        n117 = call <vilib>:"WPI_GyroReset.vi"("error in"=w173, "GyroDevRef"=w174) -> ()  [unwired: 8 in, 2 out]
      }
    }
  }
